vi "Save_odour_bottles.vi"(11 "Odour bottles in":T1(array[cluster])) -> ()   [LabVIEW 2016]
uses:
  <vilib>/Utility/xml.llb/Write to XML File(string).vi
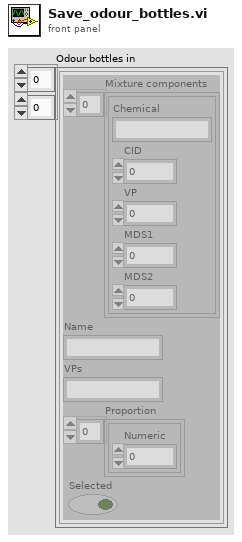
[diagram p1: front panel]
types:
  T1 = cluster{"Mixture components":cluster{"Chemical":string, "CID":i32, "VP":dbl, "MDS1":dbl, "MDS2":dbl}[], "Name":string, "VPs":string, "Proportion":cluster{"Numeric":dbl}[], "Selected":bool}[][]
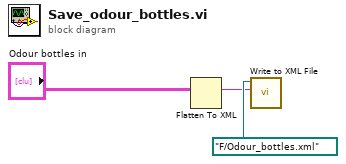
[diagram p0: block diagram]
diagram:
  n1 = Flatten To XML(anything="Odour bottles in") -> (xml string=w2:string)
  n2 = call-poly <vilib>:"Write to XML File.vi"("XML Input"=w2, "XML File Path"=path "F:/Odour_bottles.xml") -> ()  [unwired: 7 in, 3 out]
